vi "Execute.vi"(8 "error in (no error)":errorcluster, 9 "Channel Data (DBLs Only)":T3={"Inputs"={"Data to Server"=1.0}, "Outputs"={"Data from Server"=0.0}}, 10 "Real-Time System Data":T2, 11 "Configuration Data":T1={"Timeout (ms)"=100, "Server IP"="localhost", "Port"=6340}) -> (0 "error out":errorcluster, 1 "Channel Data (DBLs Only)":T3={"Inputs"={"Data to Server"=1.0}, "Outputs"={"Data from Server"=0.0}}, 2 "Real-Time System Data":T2, 3 "Configuration Data":T1={"Timeout (ms)"=100, "Server IP"="localhost", "Port"=6340})   [LabVIEW 2013, in "TCPIP Custom Device.lvlib"]
uses:
  TCPIP Custom Device.lvlib
  Real-Time System Data.ctl
  Channel Data.ctl
  Configuration Data.ctl
panel:
  # "Controls"
  # "Indicators"
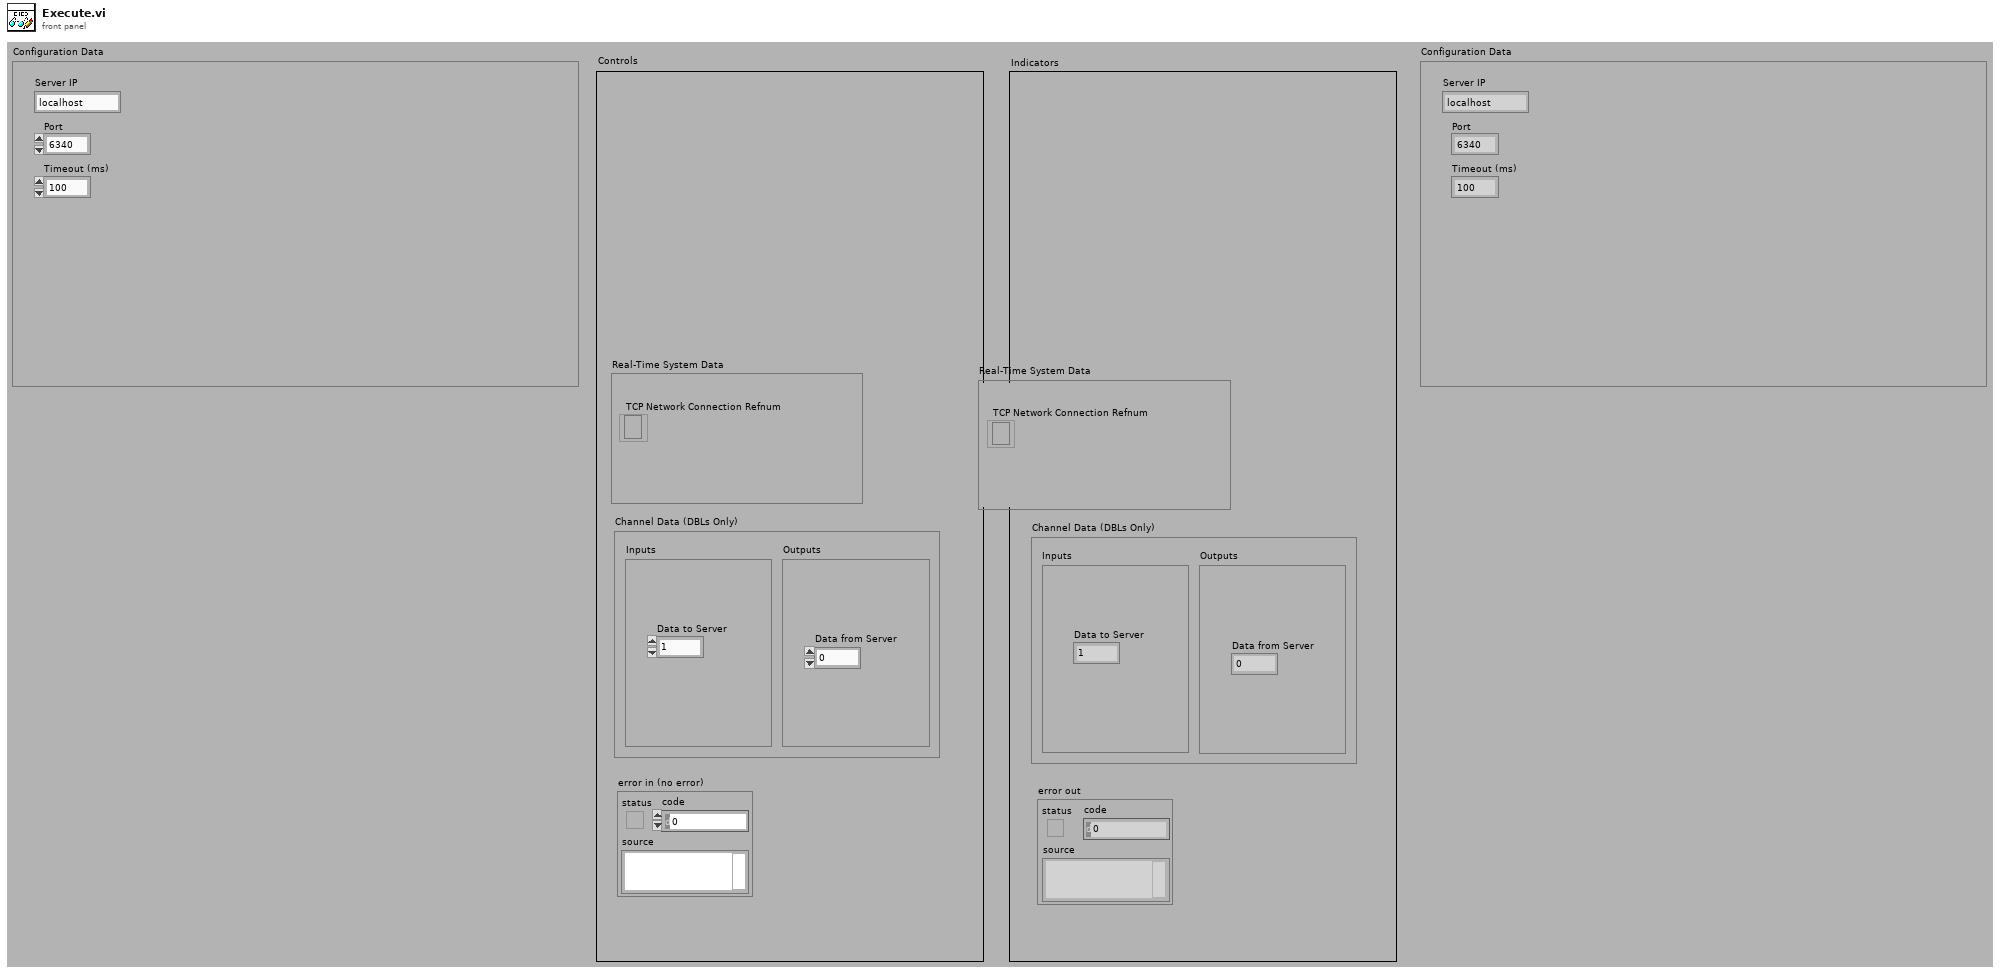
[diagram p1: front panel]
types:
  T1 = typedef "TCPIP Custom Device.lvlib/Configuration Data.ctl" = cluster{"Timeout (ms)":i32, "Server IP":string, "Port":i32}
  T2 = typedef "TCPIP Custom Device.lvlib/Real-Time System Data.ctl" = cluster{"TCP Network Connection Refnum":refnum<k5>}
  T3 = typedef "TCPIP Custom Device.lvlib/Channel Data.ctl" = cluster{"Inputs":cluster{"Data to Server":dbl}, "Outputs":cluster{"Data from Server":dbl}}
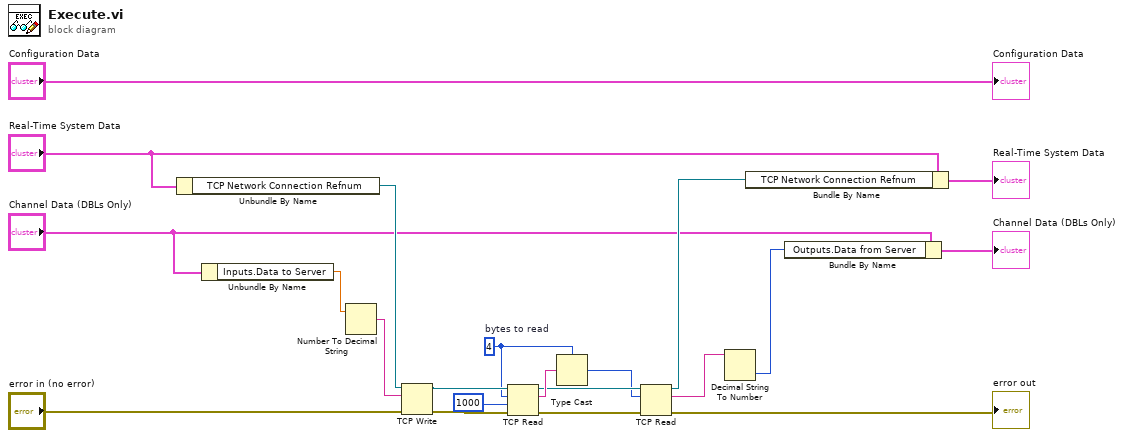
[diagram p0: block diagram]
diagram:
  w9 = 4  # bytes to read
  n1 = Unbundle By Name("Real-Time System Data") -> ("TCP Network Connection Refnum"=w18:refnum<k5>)
  n2 = Unbundle By Name("Channel Data (DBLs Only)") -> ("Inputs.Data to Server"=w16:dbl)
  n3 = Number To Decimal String(number=w16) -> (decimal integer string=w17:string)  [unwired: 1 in]
  n4 = TCP Write(connection ID=w18, data in=w17, error in (no error)="error in (no error)") -> (connection ID out=w19:refnum<k5>, error out=w15:errorcluster)  [unwired: 2 out]
  n5 = TCP Read(connection ID=w19, bytes to read=w9, error in (no error)=w15, 9:1000 ("timeout ms (25000)")) -> (connection ID out=w11:refnum<k5>, data out=w12:string, error out=w10:errorcluster)  [unwired: 1 in]
  n6 = Type Cast(type=w9, x=w12) -> (*(type *) &x=w8:i32)
  n7 = TCP Read(connection ID=w11, bytes to read=w8, error in (no error)=w10) -> (connection ID out=w20:refnum<k5>, data out=w14:string, error out=→"error out":errorcluster)  [unwired: 2 in]
  n8 = Decimal String To Number(string=w14) -> (number=w13:i32)  [unwired: 2 in, 1 out]
  n9 = Bundle By Name(cluster="Real-Time System Data", "TCP Network Connection Refnum"=w20) -> (→"Real-Time System Data":T2)
  n10 = Bundle By Name(cluster="Channel Data (DBLs Only)", "Outputs.Data from Server"=w13) -> (→"Channel Data (DBLs Only)":T3)
  "Configuration Data" <- "Configuration Data"
